vi "GetUniqueCharactersFromComics.vi"(6 "Status ref":refnum<vi>, 11 "Comics In":T1[](array[typedef]) {"Cover Price" format="$%.2g"}) -> (2 "Character URLs":string[](array[string]), 3 "Comics Out":T1[](array[typedef]) {"Cover Price" format="$%.2g"})   [LabVIEW 2022 SP3]
uses:
  TypeDefs/Comic.ctl
  TypeDefs/Character.ctl
  TypeDefs/Creator.ctl
  TypeDefs/Variant.ctl
  b97d25dd-4264-4118-ad1a-02229d48a430.vi
panel:
  out "Filtered Size":i32
  out "Raw Size":i32
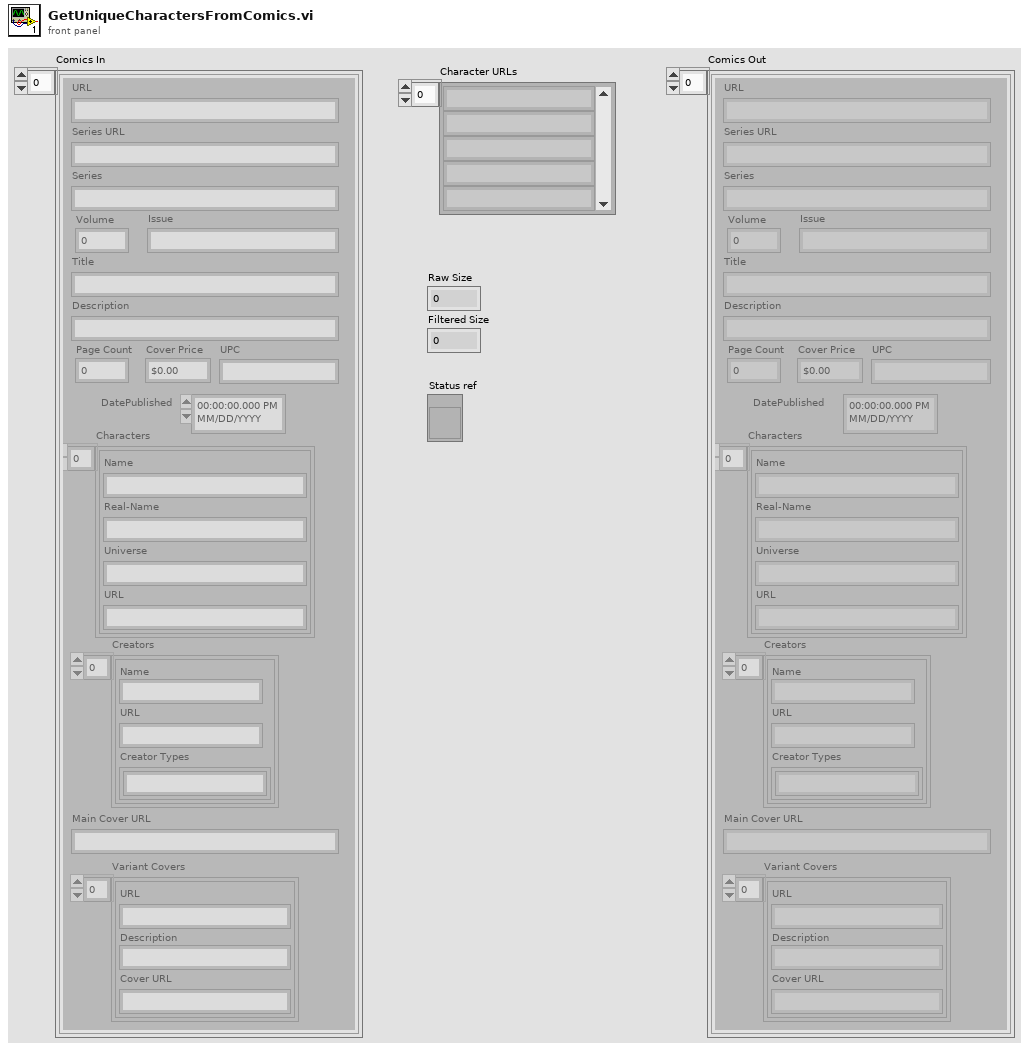
[diagram p1: front panel]
types:
  T1 = typedef "Comic.ctl" = cluster{"URL":string, "Series URL":string, "Series":string, "Volume":i32, "Issue":string, "Title":string, "Description":string, "Page Count":i32, "Cover Price":dbl, "UPC":string, "Characters":T2[], "Creators":T3[], "Main Cover URL":string, "Variant Covers":T4[], "DatePublished":timestamp}
  T2 = typedef "Character.ctl" = cluster{"Name":string, "Real-Name":string, "Universe":string, "URL":string}
  T3 = typedef "Creator.ctl" = cluster{"Name":string, "URL":string, "Creator Types":string[]}
  T4 = typedef "Variant.ctl" = cluster{"URL":string, "Description":string, "Cover URL":string}
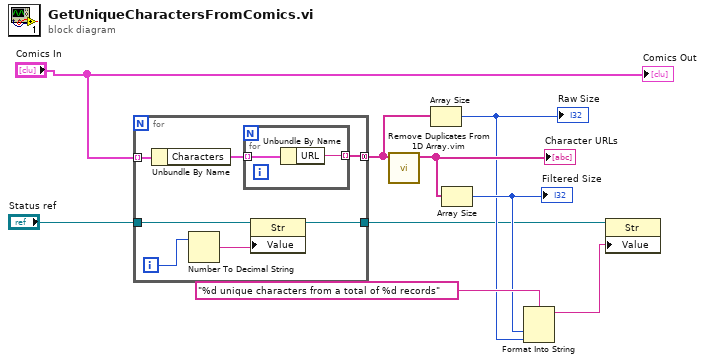
[diagram p0: block diagram]
diagram:
  n1 = for {
    tunnel: "Comics In" -> [w16] mode=indexing
    tunnel: [w10] -> w8 mode=concatenating
    tunnel: "Status ref" -> [w15]
    tunnel: [w12] -> w2
    i -> [w14]
    n2 = Unbundle By Name(w16) -> ("Characters"=w11:T2[])
    n3 = Number To Decimal String(number=w14) -> (decimal integer string=w13:string)  [unwired: 1 in]
    n4 = for {
      tunnel: w11 -> [w18] mode=indexing
      tunnel: [w17] -> w10 mode=indexing
      n5 = Unbundle By Name(w18) -> ("URL"=w17:string)
    }
    n6 = property class="Str"(reference=w15, "Value"=w13) -> (reference out=w12:refnum<vi>)  [unwired: 1 in, 1 out]
  }
  n7 = call "Remove Duplicates From 1D Array.vim"("array"=w8) -> ("array with duplicates removed"=w7:string[])  [unwired: 10 in]
  "Character URLs" <- w7
  n8 = Array Size(array=w8) -> (size(s)=w4:i32)
  "Raw Size" <- w4
  n9 = Array Size(array=w7) -> (size(s)=w5:i32)
  "Filtered Size" <- w5
  n10 = Format Into String(format string="%d unique characters from a total of %d records", w5, w4) -> (resulting string=w1:string)  [unwired: 2 in, 1 out]
  n11 = property class="Str"(reference=w2, "Value"=w1) -> ()  [unwired: 1 in, 2 out]
  "Comics Out" <- "Comics In"
